vi "vidiff ini filename.vi"() -> (3 "VIdiff INI file":string="vidiff.ini")   [LabVIEW 2016]
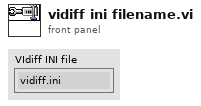
[diagram p1: front panel]
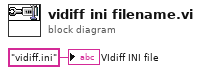
[diagram p0: block diagram]
diagram:
  "VIdiff INI file" <- "vidiff.ini"
